vi "Extra_Commands_Global.vi"() -> ()   [LabVIEW 2022 SP3]
uses:
  Controls/ExtraComandDescriptor.ctl
panel:
  in  "!Traverse Speed Factor":string="!Traverse Speed Factor"
  in  "sortPoints":string="!sortPoints"
  in  "Gas Line Name":string="!Gas Line Name"
  in  "Block Length (s)":string="!Block Length (s)"
  in  "!Offset dx;dy;dz in Model Coord":string="!Offset dx;dy;dz in Model Coord"
  in  "Suppress Route Check Errors":string="!Suppress Route Check Errors"
  in  "!3D Live Position Offset":string="!3D Live Position Offset"
  in  "!Offset dx;dy;dz in Tunnel Coord":string="!Offset dx;dy;dz in Tunnel Coord"
  in  "Trav_Profile_Plug_In":string="!Trav_Profile_Plug_In"
  in  "!Use_2D_Offset_for_Axes":string="!Use_2D_Offset_for_Axes"
  in  "!Use_Axis_Correction":string="!Use_Axis_Correction"
  in  "ExtraCommands- #NotYetImplemented":T1[][](array[typedef])=[[{"Description"="", "TriggerText"="!Puff Duration Sec", "ExampleArgument"="", "Notes"=""}], [{"Description"="", "TriggerText"="!Point Spacing ", "ExampleArgument"="", "Notes"=""}], [{"Description"="", "TriggerText"="!Work in Tunnel Coordinates", "ExampleArgument"="", "Notes"=""}], [{"Description"="", "TriggerText"="!Skip Traverse Position ", "ExampleArgument"="", "Notes"=""}], [{"Description"="", "TriggerText"="!Skip Tunnel Speed Demand", "ExampleArgument"="", "Notes"=""}], [{"Description"="", "TriggerText"="!Establish Exp Conditions (s)", "ExampleArgument"="", "Notes"=""}], [{"Description"="", "TriggerText"="!IF", "ExampleArgument"="", "Notes"=""}], [{"Description"="", "TriggerText"="!Traverse Setup", "ExampleArgument"="", "Notes"=""}], [{"Description"="", "TriggerText"="!Home", "ExampleArgument"="", "Notes"=""}], [{"Description"="", "TriggerText"="!Datum Image", "ExampleArgument"="", "Notes"=""}], [{"Description"="", "TriggerText"="!Skip Source Demand", "ExampleArgument"="", "Notes"=""}], [{"Description"="", "TriggerText"="!Not Using Source", "ExampleArgument"="", "Notes"=""}], [{"Description"="", "TriggerText"="!Repeat First Position", "ExampleArgument"="", "Notes"=""}], [{"Description"="", "TriggerText"="!Minutes Before Repeating Row", "ExampleArgument"="", "Notes"=""}], [{"Description"="", "TriggerText"="!Pause Until", "ExampleArgument"="", "Notes"=""}], [{"Description"="", "TriggerText"="!Skip if Sd Error is Below", "ExampleArgument"="", "Notes"=""}], [{"Description"="", "TriggerText"="!Add Height to Local Floor Height", "ExampleArgument"="", "Notes"=""}], [{"Description"="", "TriggerText"="!TrackStack", "ExampleArgument"="", "Notes"=""}]]
  in  "Track Object on Turntable":string="!TrackStack"
  in  "Datum Image":string="!Datum Image"
  out "If command global value":dbl
  in  "!Traverse Setup":string="!Traverse Setup"
  in  "Skip if Sd Error is Below":string="!Skip if Sd Error is Below"
  in  "Minutes Before Repeating Row":string="!Minutes Before Repeating Row"
  in  "Home":string="!Home"
  in  "Pause Until":string="!Pause Until"
  in  "If Command":string="!IF"
  in  "Skip Source Demand":string="!Skip Source Demand"
  in  "Not Using Source":string="!Not Using Source"
  in  "Repeat First Position":string="!Repeat First Position"
  in  "Skip Traverse Position Demand":string="!Skip Traverse Position Demand"
  in  "Establish Exp Conditions (s)":string="!Establish Exp Conditions (s)"
  in  "Skip Tunnel Speed Demand":string="!Skip Tunnel Speed Demand"
  in  "Work in Tunnel Coordinates":string="!Work in Tunnel Coordinates"
  in  "Point Spacing Parameters":string="!Point Spacing Parameters"
  in  "Puff Duration Sec":string="!Puff Duration Sec"
  # "#ToDo: generalise ExtraCommands into array including full description, error text etc..."
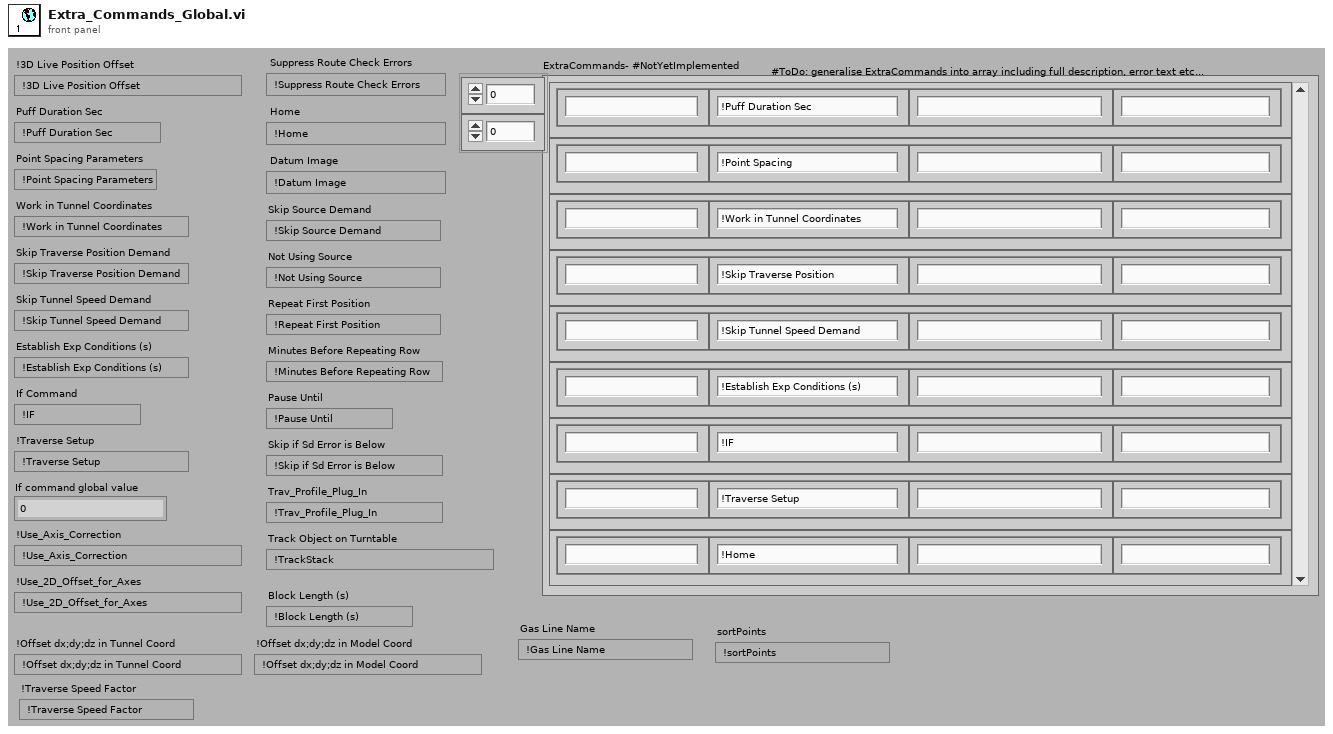
[diagram p1: front panel]
types:
  T1 = typedef "ExtraComandDescriptor.ctl" = cluster{"Description":string, "TriggerText":string, "ExampleArgument":string, "Notes":string}
diagram:
